vi "Tool_Unicode Update String.vi"(5 "Interpret as Unicode (T)":bool=TRUE, 6 "error in (no error)":errorcluster, 7 "Caption":string, 8 "String Value":string, 9 "String Control Reference":refnum<vi>) -> (0 "error out":errorcluster, 3 "String Control Reference":refnum<vi>)   [LabVIEW 2020]
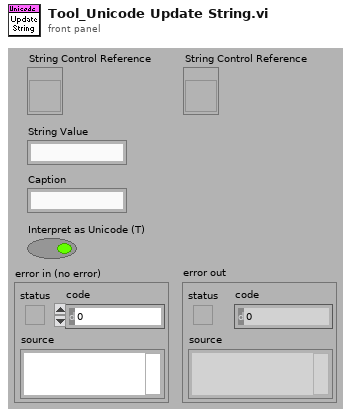
[diagram p1: front panel]
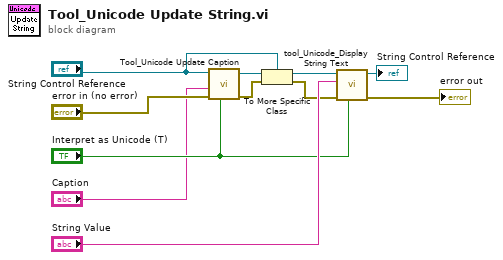
[diagram p0: block diagram]
diagram:
  n1 = call "Tool_Unicode Update Caption.vi"("Interpret as Unicode (T)"="Interpret as Unicode (T)", "error in (no error)"="error in (no error)", "Caption"="Caption", "Control Reference"="String Control Reference") -> ("error out"=w7:errorcluster, "Control Reference"=w6:refnum<vi>)  [unwired: 4 in]
  n2 = To More Specific Class(target class="String Control Reference", reference=w6, error in=w7) -> (specific class reference=w4:refnum<vi>, error out=w5:errorcluster)
  n3 = call "tool_Unicode_Display String Text.vi"("Interpret as Unicode (T)"="Interpret as Unicode (T)", "error in"=w5, "String Value"="String Value", "String Control Reference"=w4) -> ("error out"=→"error out":errorcluster, "String Control Reference"=→"String Control Reference":refnum<vi>)  [unwired: 4 in]
